vi "LabVIEW FPGA FFT.vi"() -> ()   [LabVIEW 2020]
doc: "This FPGA VI illustrates use of the FFT in a single-cycle Timed Loop (SCTL). The FFT returns results in a \"burst\" fashion, requiring several calls on average for each valid output result.\n\nThe entire data pipeline uses a handshaking protocol to ensure that no data is lost, by throttling upstream nodes if any node is not ready to receive data. If the pipeline is too slow (as determined by the host VI DMA Read loop), the Sine Wave FIFO will eventually overflow, returning Timed Out? and notifies the host UI."
uses:
  Type Definitions/Windows.ctl
  <vilib>/Platform/TimedLoop/XDataNode/timing_clust.ctl
  <vilib>/Platform/TimedLoop/XDataNode/nitl_modes.ctl
  <vilib>/Platform/TimedLoop/XDataNode/wakeup.ctl
  <vilib>/rvi/Analysis/measure/FFT/simModelSupport/niFPGA FFT Sim Properties.ctl
  <vilib>/rvi/Analysis/measure/FFT/simModelSupport/niFPGA FFT Sim Types.ctl
  <vilib>/rvi/Analysis/measure/FFT/simModelSupport/niFpgaFFTSimArithmeticProperties.ctl
  <vilib>/rvi/Analysis/measure/FFT/simModelSupport/niFpgaFFTSimDfxp.ctl
  <vilib>/fxp/LVFixedPointQuantizationPolicyTypeDef.ctl
  <vilib>/rvi/Emulation/niFpgaGetClockAttributes.vi
  <vilib>/rvi/Emulation/niFpgaSctlEmulationGetInTimedLoop.vi
  <vilib>/rvi/Emulation/niFpgaEmulationReportErrorSimple.vi
  <vilib>/rvi/DataTransferAndStorage/Container/Common/niFpgaContainerGetUniqueNameForEmu.vi
  <vilib>/rvi/DataTransferAndStorage/Container/Common/niFpgaContainerSetEmuInfo.vi
  <vilib>/rvi/eio/common/nirviEmuReportErrorAndStop.vi
  <vilib>/rvi/Emulation/niFpgaCriticalErrorInLSC.vi
  <vilib>/rvi/interface/RandomDataEmulation/niFpgaRandomDataHandleErrors.vi
  <vilib>/rvi/DataTransferAndStorage/Container/Common/niFpgaContainerExecOnDevCompGetState.vi
  <vilib>/rvi/Emulation/niFpgaEmulationIsFPGAContextNoSignature.vi
  <vilib>/rvi/errors/niFpgaSetErrorForExecOnDevCompSimple.vi
  <vilib>/rvi/FIFO/Fifo_Resource/nirvififoEmulationSetSize.vi
  <vilib>/rvi/FIFO/Fifo_Resource/nirviFifoEmulationQueueMgr.vi
  <instcachedir>/0/nirviFifoEmulationQueueMgr_E5CAEC123FF24DC58D834DCA3CDAA9B5.lvgen/nirviFifoEmulationQueueMgr_E5CAEC123FF24DC58D834DCA3CDAA9B5_002.vi
  <vilib>/rvi/FIFO/Fifo_Resource/nirvififoEmulationDetermineInputValidOut.vi
  <vilib>/rvi/FIFO/Fifo_Resource/nirvififoEmulationCreateLock.vi
  <vilib>/rvi/Emulation/niFpgaProcessEmulError.vi
  <vilib>/rvi/FIFO/Fifo_Resource/nirvififoEmulationObtainLock.vi
  <vilib>/rvi/FIFO/Fifo_Resource/nirvififoEmulationReleaseLock.vi
  <vilib>/rvi/occurrence/nirviWaitOnOccurrenceBase.vi
  <vilib>/rvi/errors/nirviReportUnexpectedCaseInternalError.vi
  <vilib>/rvi/errors/nirviReportUnexpectedCaseInternalError (U32).vi
  <vilib>/Utility/error.llb/Clear Errors.vi
  <vilib>/rvi/Analysis/measure/FFT/simModelSupport/niFpgaFFTSimModelCore.vi
  <vilib>/Platform/TimedLoop/XDataNode/XDataNode.xnode
  <vilib>/rvi/LocalResourceManager/LocalResourceManager.xnode
  <vilib>/rvi/DataTransferAndStorage/Container/XNode/niFpgaContainer.xnode
  <vilib>/rvi/interface/RandomDataEmulation/nirviRandomDataFpgaReadWriteTemplate.vi
  <vilib>/rvi/FIFO/Fifo_Resource/niFpgaFifoEmulationRefIn.vi
  <vilib>/rvi/Analysis/measure/FFT/XNode/niFpgaFFT.xnode
  <vilib>/Platform/TimedLoop/XDataNode/XDNodeRunTimeDep.lvlib
panel:
  in  "Window select":T1=enum."None"
  out "Overflow":bool
  out "Actual Sample Period (ticks)":u32
  in  "Frequency (periods/tick)":fxp<+,32,0>=0.0002500000409781933
  out "Invalid Period":bool
  in  "Requested Sample Period (ticks)":u32=1000
  # "Overview: Demonstrates the use of the LabVIEW FPGA FFT function for custom in-hardware signal processing\nRequirements: LabVIEW FPGA Module, NI-RIO\nInstructions: Run the VI"
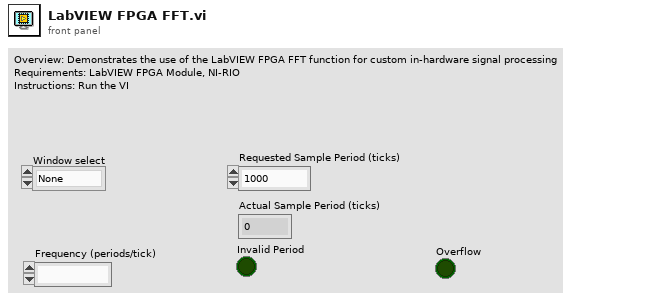
[diagram p1: front panel]
types:
  T1 = typedef "Windows.ctl" = enum16{"Hamming", "Hanning", "None"}
  T2 = typedef "XDNodeRunTimeDep.lvlib/timing_clust.ctl" = cluster{"Expected End [f-1]":u64, "Actual End [f-1]":u64, "Finished Late? [f-1]":bool, "Expected End [i-1]":u64, "Actual End [i-1]":u64, "Finished Late? [i-1]":bool, "Expected Start [i]":u64, "Actual Start [i]":u64, "Expected Start [f]":u64, "Actual Start [f]":u64, "Source Name":string, "Structure Name":string, "Period":i64, "Deadline":i64, "Offset":i64, "Start":i64, "Priority":i32, "Timeout":i32, "Mode":T3, "Wakeup Reason":T4, "Error":errorcluster, "Source Type":string, "Secondary Source Type":string, "Global End Time":u64, "Global Start Time":u64, "Frame Duration":u64, "Iteration Duration":u64, "Assigned CPU":i32, "I/O Scan Engine Mode":u32}
  T3 = typedef "XDNodeRunTimeDep.lvlib/nitl_modes.ctl" = enum32{"No Change", "Process missed periods, maintain original phase", "Discard missed periods, maintain original phase", "Process missed periods, ignore original phase", "Discard missed periods, ignore original phase"}
  T4 = typedef "XDNodeRunTimeDep.lvlib/wakeup.ctl" = enum32{"Normal", "Aborted", "Asynchronous wakeup", "Timing source error", "Timed loop error", "Timeout"}
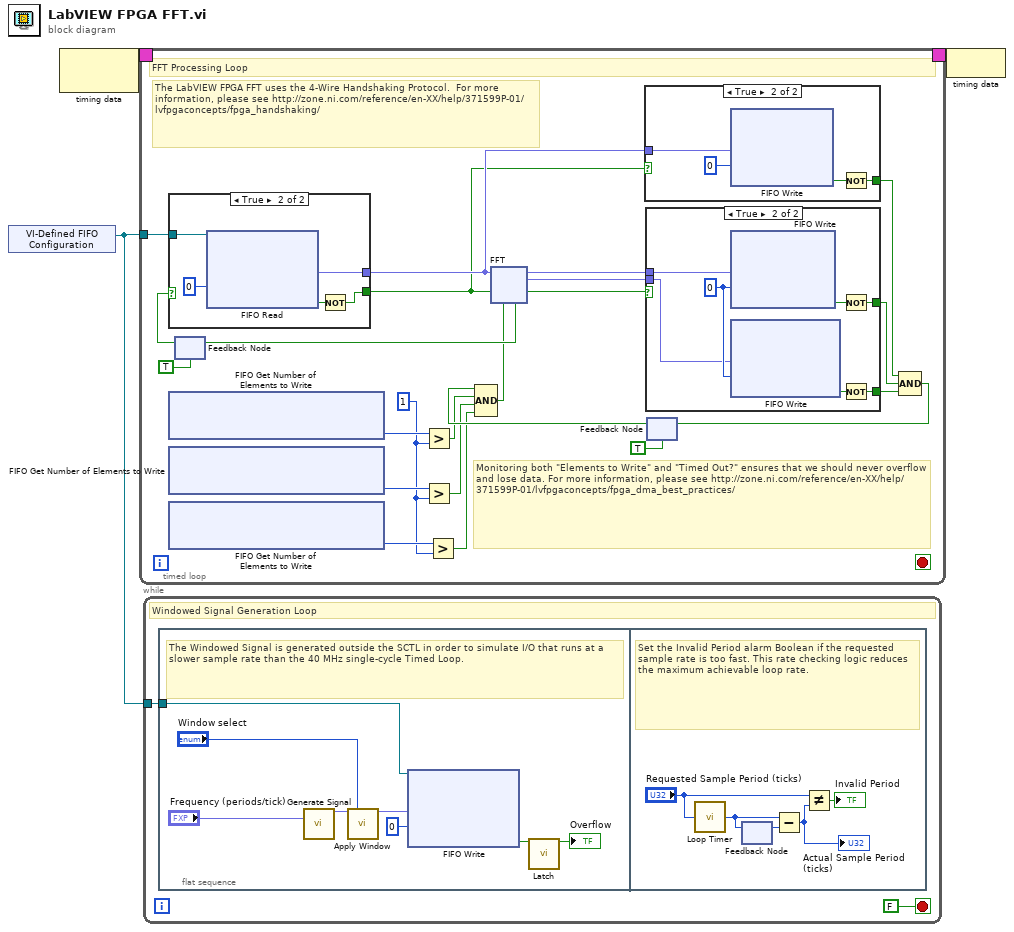
[diagram p0: block diagram]
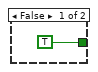
[diagram p2: hidden frame]
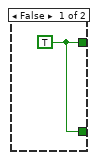
[diagram p3: hidden frame]
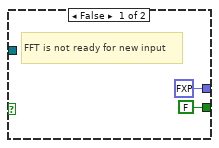
[diagram p4: hidden frame]
diagram:
  n1 = xnode "VI-Defined FIFO Configuration"() -> ("FIFO Out"=w1:refnum<k21>)
  n2 = node-c288() -> (w3:T2)  [unwired: 1 in]
  n3 = timed-loop {
    timing: w3 -> [_]
    timing-out: [_] -> w2
    tunnel: w1 -> [w22]
    stop <- _ stop-if-true
    w10 = u32 1 ("y")
    # "Monitoring both \"Elements to Write\" and \"Timed Out?\" ensures that we should never overflow and lose data. For more information, please see http://zone.ni.com/reference/en-XX/help/371599P-01/lvfpgaconcepts/fpga_dma_best_practices/"
    # "The LabVIEW FPGA FFT uses the 4-Wire Handshaking Protocol.  For more information, please see http://zone.ni.com/reference/en-XX/help/371599P-01/lvfpgaconcepts/fpga_handshaking/"
    # "FFT Processing Loop"
    n4 = xnode ("FIFO Get Number of Elements to Write")() -> ("Number of Elements to Write"=w13:u32)  [unwired: 1 in, 1 out]
    n5 = xnode ("FIFO Get Number of Elements to Write")() -> ("Number of Elements to Write"=w12:u32)  [unwired: 1 in, 1 out]
    n6 = xnode ("FIFO Get Number of Elements to Write")() -> ("Number of Elements to Write"=w11:u32)  [unwired: 1 in, 1 out]
    n7 = feedback #1(TRUE ("ready for input")) -> (w26:bool)
    n8 = case shown="True" w26 {
      tunnel: [FALSE w71] -> w23
      tunnel: [fxp<+/-,16,5> 0.0 ("Element") w72] -> w25
      tunnel: w22 -> [_ w68]
      frame False {
        # "FFT is not ready for new input"
      }
      frame True {
        n9 = xnode ("FIFO Read")("Timeout"=0, "FIFO In"=w68) -> ("Element"=w72:fxp<+/-,16,5>, "Timed Out?"=w70:bool)  [unwired: 1 out]
        n10 = Not(x=w70) -> (.not. x?=w71:bool)
      }
    }
    n11 = Greater?(x=w13, y=w10) -> (0:w7:bool)
    n12 = Greater?(x=w12, y=w10) -> (0:w6:bool)
    n13 = Greater?(x=w11, y=w10) -> (0:w5:bool)
    n14 = case shown="True" w23 {
      tunnel: w25 -> [_ w54]
      tunnel: [TRUE ("Timed Out?") w55] -> w18
      frame False {
      }
      frame True {
        n15 = xnode ("FIFO Write")("Element"=w54, "Timeout"=0) -> ("Timed Out?"=w56:bool)  [unwired: 1 in, 1 out]
        n16 = Not(x=w56) -> (.not. x?=w55:bool)
      }
    }
    n17 = feedback #2(TRUE) -> (w8:bool)
    n18 = Compound Arithmetic op=AND(w8, w7, w6, w5) -> (w9:bool)
    n19 = xnode "FFT"("real data in"=w25, "input valid"=w23, "ready for output"=w9) -> ("ready for input"=w24:bool, "real data out"=w21:fxp<+/-,25,14>, "imaginary data out"=w20:fxp<+/-,25,14>, "output valid"=w19:bool)  [unwired: 2 in, 1 out]
    n20 = feedback-in #1(w24) -> ()
    n21 = case shown="True" w19 {
      tunnel: w21 -> [_ w60]
      tunnel: w20 -> [_ w59]
      tunnel: [w58 w62] -> w17
      tunnel: [w58 w61] -> w16
      frame False {
        w58 = TRUE ("Timed Out?")
      }
      frame True {
        w65 = 0 ("Timeout")
        n22 = xnode ("FIFO Write")("Element"=w60, "Timeout"=w65) -> ("Timed Out?"=w64:bool)  [unwired: 1 in, 1 out]
        n23 = xnode ("FIFO Write")("Element"=w59, "Timeout"=w65) -> ("Timed Out?"=w63:bool)  [unwired: 1 in, 1 out]
        n24 = Not(x=w64) -> (.not. x?=w62:bool)
        n25 = Not(x=w63) -> (.not. x?=w61:bool)
      }
    }
    n26 = Compound Arithmetic op=AND(w18, w17, w16) -> (w15:bool)
    n27 = feedback-in #2(w15) -> ()
  }
  n28 = while {
    tunnel: w1 -> [w76]
    stop <- FALSE stop-if-true
    # "Windowed Signal Generation Loop"
    n29 = flat-sequence {
      tunnel: w76 -> [w80]
      frame #0 {
        # "The Windowed Signal is generated outside the SCTL in order to simulate I/O that runs at a slower sample rate than the 40 MHz single-cycle Timed Loop."
        n30 = call "Generate Signal.vi"("frequency (periods/tick)"="Frequency (periods/tick)") -> ("signal"=w81:fxp<+/-,16,5>)  [unwired: 14 in]
        n31 = call "Apply Window.vi"("Signal In"=w81, "Window select"="Window select") -> ("Windowed Signal Out"=w82:fxp<+/-,16,5>)  [unwired: 13 in]
        n32 = xnode ("FIFO Write")("Element"=w82, "Timeout"=0, "FIFO In"=w80) -> ("Timed Out?"=w79:bool)  [unwired: 1 out]
        n33 = call "Latch.vi"("Input"=w79) -> ("Output"=→"Overflow":bool)  [unwired: 14 in]
      }
      frame #1 {
        # "Set the Invalid Period alarm Boolean if the requested sample rate is too fast. This rate checking logic reduces the maximum achievable loop rate."
        n34 = call "Loop Timer"("Count(Ticks)"="Requested Sample Period (ticks)") -> ("Tick Count(Ticks)"=w85:u32)
        n35 = feedback #3() -> (w86:u32)  [unwired: 1 in]
        n36 = feedback-in #3(w85) -> ()
        n37 = Subtract(x=w85, y=w86) -> (x-y=w89:u32)
        "Actual Sample Period (ticks)" <- w89
        n38 = Not Equal?(x="Requested Sample Period (ticks)", y=w89) -> (x != y?=→"Invalid Period":bool)
      }
    }
  }
  n39 = node-c288(w2) -> ()
